vi "ReadStrains.vi"() -> ()   [LabVIEW 2017]
doc: "I. Description:\nThis example demonstrates how to make continuous, hardware-timed temperature measurement using a thermocouple.\n\nII. Instructions for Running:\n1. Specify the Physical Channel where you have connected the thermocouple.\n2. Enter the Minimum and Maximum temperature values in degrees C you expect to measure. A smaller range will allow a more accurate measurement.\n3. Enter the scan rate at which you want to run the acquisition.\n4. Specify the type of thermocouple you are using.\n5. Thermocouple measurements require cold-junction compensation (CJC) to correctly scale them. Specify the source of your cold-junction compensation.\n6. If your CJC source is \"Internal\", skip the rest of the steps.\n7. If your CJC source is \"Constant Value\", specify the value (usually room temperature) in degrees C.\n8. If your CJC source is \"Channel\", specify the CJC Channel name. \n9. Specify the appropriate Auto Zero Mode. See your device's hardware manual to find out if your device supports this attribute.\n\nIII. Block Diagram Steps:\n1. Create a Thermocouple (TC) temperature measurement channel.\n2. Get all the channels in the task.\n3. Convert channel(s) array to a comma-delimited channel string.\n4. This attribute is set to compensate for input offset errors. May not be supported by all devices*.\n5. Call the Timing VI to specify the hardware timing parameters. Use device's internal clock, continuous mode acquisition and the sample rate specified by the user.\n6. Call the Start VI to program and start the acquisition.\n7. Read N samples and plot it. By default, the Read VI reads all available samples, but you can specify how many samples to read at a time and the timeout value. Continue reading data until the stop button is pressed or an error occurs. \n8. Call the Clear Task VI to clear the Task.\n9. Use the popup dialog box to display an error if any.\n\n* If your device does not support Auto Zero Mode bypass Step 2, 3, and 4.\n\nIV. I/O Connections Overview:\nConnect your thermocouple to the terminals corresponding to the Physical Channel I/O Control value."
uses:
  <vilib>/Utility/error.llb/DialogType.ctl
  <vilib>/DAQmx/read.llb/DAQmx Read (Analog 1D Wfm NChan NSamp).vi
  <vilib>/Analysis/baseanly.llb/Mean (DBL).vi
  <vilib>/Waveform/WDTOps.llb/WDT Index Channel DBL.vi
  <vilib>/DAQmx/create/channels.llb/DAQmx Create Channel (AI-Voltage-Basic).vi
  <vilib>/DAQmx/configure/timing.llb/DAQmx Timing (Sample Clock).vi
  <vilib>/DAQmx/miscellaneous.llb/DAQmx Fill In Error Info.vi
  <vilib>/Analysis/NI_AALBase.lvlib
  <vilib>/ptbypt/NI_PtbyPt.lvlib
  <vilib>/Utility/miscctls.llb/LVRowAndColumnTypeDef.ctl
panel:
  in  "Data Tag":dbl=99.0 format="%.2p"
  out "Load Cell Min Peak":dbl format="%0.2f"
  out "Load Cell Max Peak":dbl format="%0.2f"
  in  "Stop":bool
  in  "Color Box":u32(colorbox)=16448250
  out "Results":i32[](listbox)
  in  "num_chans":i32=5
  out "TRQ_2SPD_OT (N·m)":dbl=-0.01305389404296875 format="%0.3f"
  out "Power_OT (W)":dbl=-4.779110606064606 format="%.2f"
  out "rpm_out/rpm_in":dbl=-8.382425226893735e-05 format="%.3g"
  out "AI Consumer Iterations":i32=456
  in  "path":path=path "D:/LabView Data"
  out "P2 - P1":dbl=2.2560862731933593 format="%.3f"
  out "Recorded Blocks":dbl=456.0
  in  "Force Record":bool caption="Force Record Enable"
  out "data 2":waveform(dbl)[](array[waveform])=[{"t0"=timestamp(3680889355.4831715 s since 1904-01-01), "dt"=0.001, "Y"=[-0.10400045911486416, -0.1030272812082663, -0.10335167384374958, -0.1030272812082663, -0.1030272812082663, -0.10270288857283233, -0.1030272812082663, -0.10270288857283233, -0.1030272812082663, -0.10367606647928221, -0.10335167384374958, -0.10367606647928221, -0.10367606647928221, -0.10367606647928221, -0.1072443854734039, -0.10237849593744763, -0.1030272812082663, -0.10270288857283233, -0.10432485175049552, -0.10367606647928221, -0.1030272812082663, -0.10335167384374958, -0.101729710666826, -0.10335167384374958, -0.10270288857283233, -0.1030272812082663, -0.10270288857283233, -0.1020541033021122, -0.10367606647928221, -0.10432485175049552, -0.10367606647928221, -0.10432485175049552, -0.10270288857283233, -0.10464924438617626, -0.10400045911486416, -0.10367606647928221, -0.10270288857283233, -0.10335167384374958, -0.1056224222935152, -0.10432485175049552, -0.10335167384374958, -0.1030272812082663, -0.10400045911486416, -0.1030272812082663, -0.10497363702190646, -0.10432485175049552, -0.10594681492939385, -0.09783699904722266, -0.10270288857283233, -0.10270288857283233, -0.10270288857283233, -0.10270288857283233, -0.10367606647928221, -0.10367606647928221, -0.10367606647928221, -0.10335167384374958, -0.10367606647928221, -0.10335167384374958, -0.10335167384374958, -0.1030272812082663, -0.10335167384374958, -0.10367606647928221, -0.10432485175049552, -0.10367606647928221, -0.10237849593744763, -0.10432485175049552, -0.1030272812082663, -0.10432485175049552, -0.10400045911486416, -0.10335167384374958, -0.10432485175049552, -0.101729710666826, -0.10335167384374958, -0.1030272812082663, -0.1020541033021122, -0.1030272812082663, -0.10270288857283233, -0.10400045911486416, -0.10432485175049552, -0.10627120756532199, -0.10367606647928221, -0.10400045911486416, -0.10237849593744763, -0.10432485175049552, -0.10367606647928221, -0.10367606647928221, -0.10237849593744763, -0.10400045911486416, -0.10756877810953042, -0.10400045911486416, -0.10237849593744763, -0.1030272812082663, -0.10270288857283233, -0.10335167384374958, -0.10335167384374958, -0.10432485175049552, -0.101729710666826, -0.10237849593744763, -0.1030272812082663, -0.10335167384374958, -0.10270288857283233, -0.10367606647928221, -0.10367606647928221, -0.10335167384374958, -0.1030272812082663, -0.10627120756532199, -0.1030272812082663, -0.10335167384374958, -0.10335167384374958, -0.1030272812082663, -0.10335167384374958, -0.1030272812082663, -0.10367606647928221, -0.10367606647928221, -0.1020541033021122, -0.10335167384374958, -0.1030272812082663, -0.10335167384374958, -0.10335167384374958, -0.10335167384374958, -0.10335167384374958, -0.10464924438617626, -0.101729710666826, -0.10270288857283233, -0.10270288857283233, -0.10270288857283233, -0.1030272812082663, -0.10270288857283233, -0.10497363702190646, -0.10756877810953042, -0.10400045911486416, -0.1030272812082663, -0.1030272812082663, -0.10367606647928221, -0.10335167384374958, -0.10400045911486416, -0.10367606647928221, -0.10432485175049552, -0.10627120756532199, -0.10497363702190646, -0.10335167384374958, -0.10367606647928221, -0.1030272812082663, -0.10335167384374958, -0.10400045911486416, -0.10335167384374958, -0.1095151339273331, -0.10432485175049552, -0.10335167384374958, -0.10237849593744763, -0.10335167384374958, -0.1030272812082663, -0.10432485175049552, -0.10270288857283233, -0.1030272812082663, -0.10756877810953042, -0.10270288857283233, -0.101729710666826, -0.10270288857283233, -0.1030272812082663, -0.10367606647928221, -0.10497363702190646, -0.10367606647928221, -0.1030272812082663, -0.1030272812082663, -0.10400045911486416, -0.10270288857283233, -0.10335167384374958, -0.1030272812082663, -0.10367606647928221, -0.10400045911486416, -0.09881017695146153, -0.101405318031589, -0.10270288857283233, -0.10270288857283233, -0.10367606647928221, -0.10400045911486416, -0.10367606647928221, -0.10367606647928221, -0.10627120756532199, -0.10367606647928221, -0.10367606647928221, -0.10270288857283233, -0.10237849593744763, -0.10464924438617626, -0.1030272812082663, -0.1030272812082663, -0.10335167384374958, -0.10627120756532199, -0.10464924438617626, -0.1030272812082663, -0.10270288857283233, -0.10270288857283233, -0.1030272812082663, -0.10367606647928221, -0.10400045911486416, -0.10075653276126252, -0.10400045911486416, -0.10270288857283233, -0.10335167384374958], "attributes"=variant("NI_ChannelName"=variant(string "Dev1/ai0"), "NI_UnitDescription"=variant(string "Volts"))}, {"t0"=timestamp(3680889355.4831853 s since 1904-01-01), "dt"=0.001, "Y"=[-0.090375968462633, -0.08972718319562067, -0.09005157582910267, -0.08972718319562067, -0.09005157582910267, -0.09005157582910267, -0.09005157582910267, -0.08972718319562067, -0.08972718319562067, -0.09005157582910267, -0.090375968462633, -0.09005157582910267, -0.090375968462633, -0.09070036109621166, -0.09297110953261792, -0.09102475372983868, -0.09070036109621166, -0.090375968462633, -0.09070036109621166, -0.09102475372983868, -0.090375968462633, -0.09005157582910267, -0.08940279056218697, -0.09005157582910267, -0.08972718319562067, -0.09005157582910267, -0.09005157582910267, -0.08940279056218697, -0.09005157582910267, -0.09070036109621166, -0.090375968462633, -0.09102475372983868, -0.090375968462633, -0.090375968462633, -0.09005157582910267, -0.09070036109621166, -0.09005157582910267, -0.09005157582910267, -0.09199793163101021, -0.0913491463635141, -0.09102475372983868, -0.090375968462633, -0.09070036109621166, -0.090375968462633, -0.09102475372983868, -0.0913491463635141, -0.09199793163101021, -0.08778082739574193, -0.08907839792880154, -0.08907839792880154, -0.08907839792880154, -0.08972718319562067, -0.090375968462633, -0.090375968462633, -0.09070036109621166, -0.09005157582910267, -0.09005157582910267, -0.090375968462633, -0.09005157582910267, -0.09005157582910267, -0.090375968462633, -0.09070036109621166, -0.09102475372983868, -0.09070036109621166, -0.090375968462633, -0.09070036109621166, -0.09005157582910267, -0.09070036109621166, -0.09070036109621166, -0.090375968462633, -0.09070036109621166, -0.08972718319562067, -0.090375968462633, -0.090375968462633, -0.08972718319562067, -0.09005157582910267, -0.08972718319562067, -0.09070036109621166, -0.09102475372983868, -0.09199793163101021, -0.09167353899723793, -0.09102475372983868, -0.090375968462633, -0.090375968462633, -0.090375968462633, -0.090375968462633, -0.08972718319562067, -0.090375968462633, -0.09264671689870017, -0.0913491463635141, -0.090375968462633, -0.090375968462633, -0.09005157582910267, -0.090375968462633, -0.09005157582910267, -0.09102475372983868, -0.08972718319562067, -0.08940279056218697, -0.09005157582910267, -0.09005157582910267, -0.08972718319562067, -0.08972718319562067, -0.09005157582910267, -0.09005157582910267, -0.090375968462633, -0.09167353899723793, -0.09070036109621166, -0.090375968462633, -0.090375968462633, -0.090375968462633, -0.090375968462633, -0.090375968462633, -0.09070036109621166, -0.09070036109621166, -0.09005157582910267, -0.08972718319562067, -0.08972718319562067, -0.08972718319562067, -0.08972718319562067, -0.090375968462633, -0.09005157582910267, -0.09102475372983868, -0.09005157582910267, -0.08972718319562067, -0.08972718319562067, -0.08972718319562067, -0.09005157582910267, -0.09005157582910267, -0.09070036109621166, -0.09264671689870017, -0.09167353899723793, -0.09102475372983868, -0.09005157582910267, -0.090375968462633, -0.09005157582910267, -0.09070036109621166, -0.090375968462633, -0.09070036109621166, -0.09167353899723793, -0.09232232426483095, -0.09102475372983868, -0.09070036109621166, -0.090375968462633, -0.09070036109621166, -0.09102475372983868, -0.09102475372983868, -0.09394428743466249, -0.09232232426483095, -0.0913491463635141, -0.09070036109621166, -0.090375968462633, -0.090375968462633, -0.09102475372983868, -0.09005157582910267, -0.09005157582910267, -0.09232232426483095, -0.0913491463635141, -0.09005157582910267, -0.09005157582910267, -0.08972718319562067, -0.090375968462633, -0.0913491463635141, -0.09070036109621166, -0.090375968462633, -0.09005157582910267, -0.09005157582910267, -0.09005157582910267, -0.09005157582910267, -0.08972718319562067, -0.09070036109621166, -0.09070036109621166, -0.08842961266217535, -0.08810522002893456, -0.08907839792880154, -0.08940279056218697, -0.09005157582910267, -0.09070036109621166, -0.09070036109621166, -0.090375968462633, -0.0913491463635141, -0.09102475372983868, -0.09070036109621166, -0.09005157582910267, -0.08972718319562067, -0.09070036109621166, -0.09005157582910267, -0.09005157582910267, -0.09005157582910267, -0.09199793163101021, -0.0913491463635141, -0.09102475372983868, -0.090375968462633, -0.09005157582910267, -0.09005157582910267, -0.090375968462633, -0.09070036109621166, -0.08907839792880154, -0.09005157582910267, -0.090375968462633, -0.09070036109621166], "attributes"=variant("NI_ChannelName"=variant(string "Dev1/ai1"), "NI_UnitDescription"=variant(string "Volts"))}, {"t0"=timestamp(3680889355.483199 s since 1904-01-01), "dt"=0.001, "Y"=[-0.1030272812082663, -0.1030272812082663, -0.10270288857283233, -0.10237849593744763, -0.10270288857283233, -0.10335167384374958, -0.10335167384374958, -0.10367606647928221, -0.10400045911486416, -0.10400045911486416, -0.10400045911486416, -0.10400045911486416, -0.10400045911486416, -0.10400045911486416, -0.10464924438617626, -0.10464924438617626, -0.10432485175049552, -0.10367606647928221, -0.10335167384374958, -0.10335167384374958, -0.10400045911486416, -0.10400045911486416, -0.10367606647928221, -0.10367606647928221, -0.10367606647928221, -0.10367606647928221, -0.10400045911486416, -0.10400045911486416, -0.10367606647928221, -0.10400045911486416, -0.10529802965768609, -0.10367606647928221, -0.10335167384374958, -0.1030272812082663, -0.10367606647928221, -0.10335167384374958, -0.10335167384374958, -0.10400045911486416, -0.10400045911486416, -0.10432485175049552, -0.10464924438617626, -0.10432485175049552, -0.10497363702190646, -0.10432485175049552, -0.10529802965768609, -0.10432485175049552, -0.10497363702190646, -0.10400045911486416, -0.1030272812082663, -0.1030272812082663, -0.10270288857283233, -0.10237849593744763, -0.10237849593744763, -0.1030272812082663, -0.1030272812082663, -0.10367606647928221, -0.10367606647928221, -0.10400045911486416, -0.10400045911486416, -0.10464924438617626, -0.10464924438617626, -0.10464924438617626, -0.10400045911486416, -0.10432485175049552, -0.10400045911486416, -0.10400045911486416, -0.10335167384374958, -0.10335167384374958, -0.10335167384374958, -0.1030272812082663, -0.10367606647928221, -0.10400045911486416, -0.1030272812082663, -0.10367606647928221, -0.10367606647928221, -0.10400045911486416, -0.10367606647928221, -0.10497363702190646, -0.10432485175049552, -0.10529802965768609, -0.10432485175049552, -0.10464924438617626, -0.10400045911486416, -0.10335167384374958, -0.10335167384374958, -0.10367606647928221, -0.10335167384374958, -0.10400045911486416, -0.10400045911486416, -0.10464924438617626, -0.10432485175049552, -0.10497363702190646, -0.10432485175049552, -0.10432485175049552, -0.10464924438617626, -0.10400045911486416, -0.10400045911486416, -0.10400045911486416, -0.10335167384374958, -0.10335167384374958, -0.1030272812082663, -0.1030272812082663, -0.1030272812082663, -0.10270288857283233, -0.1030272812082663, -0.10367606647928221, -0.10367606647928221, -0.10400045911486416, -0.10400045911486416, -0.10432485175049552, -0.10464924438617626, -0.10400045911486416, -0.10400045911486416, -0.10432485175049552, -0.10367606647928221, -0.10335167384374958, -0.10335167384374958, -0.1030272812082663, -0.10335167384374958, -0.10270288857283233, -0.10270288857283233, -0.10367606647928221, -0.10400045911486416, -0.10367606647928221, -0.10432485175049552, -0.10432485175049552, -0.10335167384374958, -0.10432485175049552, -0.10464924438617626, -0.1056224222935152, -0.10464924438617626, -0.10464924438617626, -0.10400045911486416, -0.10335167384374958, -0.10335167384374958, -0.10335167384374958, -0.10270288857283233, -0.10367606647928221, -0.10400045911486416, -0.10464924438617626, -0.10497363702190646, -0.10497363702190646, -0.10497363702190646, -0.10400045911486416, -0.10529802965768609, -0.10464924438617626, -0.1056224222935152, -0.1056224222935152, -0.10464924438617626, -0.10497363702190646, -0.10432485175049552, -0.10464924438617626, -0.10367606647928221, -0.10335167384374958, -0.10367606647928221, -0.10464924438617626, -0.10432485175049552, -0.10432485175049552, -0.10432485175049552, -0.10400045911486416, -0.10400045911486416, -0.10464924438617626, -0.10432485175049552, -0.10464924438617626, -0.10367606647928221, -0.10335167384374958, -0.1030272812082663, -0.10335167384374958, -0.10335167384374958, -0.10335167384374958, -0.10367606647928221, -0.1030272812082663, -0.1030272812082663, -0.10270288857283233, -0.10335167384374958, -0.10270288857283233, -0.10335167384374958, -0.10367606647928221, -0.10432485175049552, -0.10432485175049552, -0.10497363702190646, -0.10432485175049552, -0.10367606647928221, -0.10335167384374958, -0.10432485175049552, -0.10335167384374958, -0.10335167384374958, -0.10335167384374958, -0.10400045911486416, -0.10432485175049552, -0.10464924438617626, -0.10464924438617626, -0.10367606647928221, -0.10400045911486416, -0.10464924438617626, -0.10400045911486416, -0.10367606647928221, -0.10432485175049552, -0.10335167384374958, -0.10270288857283233], "attributes"=variant("NI_ChannelName"=variant(string "Dev1/ai2"), "NI_UnitDescription"=variant(string "Volts"))}, {"t0"=timestamp(3680889355.4832134 s since 1904-01-01), "dt"=0.001, "Y"=[9.970761347134479, 9.980493438515435, 10.057052580026493, 10.050240112411151, 10.024287857756553, 9.963948883552924, 10.009689716548086, 9.985683887516803, 9.9600560473629, 9.977573811033155, 9.974654183609161, 9.938645450165463, 9.976276198837517, 9.89614866799873, 9.958758435322546, 9.986657096725082, 10.014880166587908, 10.06808229017756, 10.063216241478031, 10.057052580026493, 10.042454435528043, 10.031100324154862, 10.03207353366638, 10.014880166587908, 9.993793964450594, 10.021043826250418, 9.967841719846424, 9.942538285787142, 9.947728733443315, 9.958434032314253, 9.952270375293104, 9.973356571439426, 10.001904041834917, 10.023963454602686, 9.984710678315004, 10.021368229397778, 10.057701386482737, 10.020395019957865, 10.040832419563271, 10.016502182263276, 9.995415979891405, 9.967517316818013, 9.966868510763346, 9.953892390273543, 9.919181273604169, 9.97173455624344, 9.920154482371043, 9.957785226299821, 9.969139331967257, 10.004499266693117, 9.996064786072774, 9.987305902867535, 10.059972209102451, 10.035966371777608, 10.032722340011015, 10.057376983254251, 10.022017035694667, 9.998011204634192, 9.979844632403223, 9.942862688760275, 9.925344929236438, 9.91723485608973, 9.96200246544498, 9.92891336156266, 9.980493438515435, 9.995415979891405, 10.006445685367076, 10.03207353366638, 10.04180562913996, 10.087870889907263, 10.03499316224003, 10.053159741349983, 9.93637462943381, 10.006121282252945, 9.980169035458967, 10.00352605736588, 9.965570898662637, 9.928264555678723, 9.949350748373524, 9.960704853387385, 9.945133509592281, 9.972707765358873, 9.99963322012187, 10.022017035694667, 10.052186531697178, 10.0512133220509, 10.06126982204397, 10.038237194057304, 10.040832419563271, 10.035966371777608, 10.00255284804514, 10.000606429423135, 9.929562167449461, 9.968814928935972, 9.933779405783481, 9.966219704711555, 9.937347838314507, 9.958758435322546, 9.976600601885348, 10.007418894713798, 10.036939581321704, 10.024287857756553, 10.052186531697178, 10.040832419563271, 10.033695549533391, 10.043752048312902, 10.017475391677165, 9.976925004933896, 9.972707765358873, 9.963948883552924, 9.95356798727602, 9.930535376285032, 9.987630305939843, 9.942213882814727, 9.978547020187436, 9.984386275249179, 9.99768680153882, 10.062243031757733, 10.047320483531054, 10.051862128481027, 10.02169263254586, 10.042454435528043, 9.96427328657343, 10.018773004239138, 9.977898214083861, 9.98146664768915, 9.97303216839879, 9.951297166313452, 9.938645450165463, 9.957136420288261, 9.937023435353558, 9.973356571439426, 9.992171949027805, 9.993469561364593, 10.02915390515136, 10.057701386482737, 10.071975129254877, 10.03629077495825, 10.053159741349983, 10.038237194057304, 10.01844860109756, 9.970112541065435, 9.933130599878064, 9.98081784157262, 9.942862688760275, 9.972058959281199, 9.943511494708691, 9.951621569305953, 9.978871423240303, 9.998011204634192, 9.976925004933896, 9.983413066056023, 10.069379903191706, 10.04537406431028, 10.04991570919935, 10.04796928994378, 10.015528972855886, 10.014231360322817, 9.997362398444167, 9.954541196270744, 9.95032395734026, 9.919830079448037, 9.96200246544498, 9.952919181283127, 9.972058959281199, 9.992820755194758, 10.029802711482967, 10.055754967122715, 10.006445685367076, 10.051862128481027, 10.02363905144954, 10.038561597243016, 10.057701386482737, 10.014880166587908, 9.972058959281199, 9.959082838331556, 10.037588387688057, 9.927291346858187, 9.929886570393936, 9.926642540981407, 9.92339851164045, 9.960380450374785, 9.987954709012872, 10.017475391677165, 10.019097407381437, 10.058025789711948, 10.067109080424581, 10.02688308301353, 9.956812017283559, 10.046347273917407, 10.015204569721535, 9.986008290585508, 9.950648360330606, 9.98146664768915, 9.923074108710292, 9.96524649563926, 9.932481793975509, 9.956487614279574, 9.983088662993078, 10.021368229397778], "attributes"=variant("NI_ChannelName"=variant(string "Dev1/ai3"), "NI_UnitDescription"=variant(string "Volts"))}]
  out "Power_IN (W)":dbl=0.0005711775684961294 format="%.2g"
  out "TRQ_2SPD_DRVLN_OT (N·m)":dbl=-0.018612060546874976 format="%0.3f"
  out "Waveform Chart":waveform(dbl)[](graph)=[{"t0"=timestamp(3680889355.4831715 s since 1904-01-01), "dt"=0.01, "Y"=[-20.631407652497842, -20.75467685406648, -20.59896838896825, -20.780628264870508, -20.637895505396592, -20.663846916046168, -20.728725443162563, -20.696286179664597, -20.793603970347206, -20.59248053625661, -20.709261885055327, -20.644383357919143, -20.722237590555686, -20.806579675725974, -20.806579675853744, -20.683310474277953, -20.70277403231996, -20.618431947232246, -20.748189001336023, -20.598968388981042], "attributes"=variant("NI_ChannelName"=variant(string "HS_LOADCELL_A_LBF"), "NI_UnitDescription"=variant(string "lbf"))}, {"t0"=timestamp(3680889355.4831853 s since 1904-01-01), "dt"=0.01, "Y"=[-17.99085160781258, -18.16602362995864, -17.99733946048705, -18.12709651391563, -18.055730134580486, -18.01680301849887, -18.114120808557974, -18.088169397890056, -18.16602362996153, -18.029778723839122, -18.068705839868564, -18.029778723838152, -18.075193692560465, -18.1789993353008, -18.26334142007583, -18.107632955909622, -18.068705839864695, -17.977875902519663, -18.114120808576352, -18.05573013452541], "attributes"=variant("NI_ChannelName"=variant(string "HS_LOADCELL_B_LBF"), "NI_UnitDescription"=variant(string "lbf"))}, {"t0"=timestamp(3680889355.483199 s since 1904-01-01), "dt"=0.01, "Y"=[-0.10322191678961545, -0.1040004591149086, -0.10383826279707317, -0.10380582353359895, -0.10429241248705587, -0.10335167384387292, -0.10387070206069556, -0.10403289837852114, -0.10393558058779713, -0.10413021616916611, -0.10344899163446859, -0.10364362721580296, -0.10406533764211885, -0.10383826279716202, -0.1049736370219559, -0.10413021616915127, -0.10377338427002589, -0.10341655237092517, -0.10390314132425375, -0.1039680198513899], "attributes"=variant("NI_ChannelName"=variant(string "HS_2210_STRAIN_B_VOLTS"), "NI_UnitDescription"=variant(string "V"))}, {"t0"=timestamp(3680889355.4832134 s since 1904-01-01), "dt"=0.01, "Y"=[9.997978768185797, 9.993437131092849, 9.995188902202935, 10.009300435915007, 9.962618833492515, 10.0112144154578, 9.987760076882132, 9.981823496420388, 10.021919719195791, 9.968166125458495, 10.016275103370784, 9.993599329306088, 9.982666942582545, 10.01825396484399, 9.96894469235443, 10.015464096552865, 9.989382089044614, 9.988733284529754, 10.006348371443773, 9.97150747733223], "attributes"=variant("NI_ChannelName"=variant(string "HS_2210_EXC_VOLTS"), "NI_UnitDescription"=variant(string "V"))}]
  in  "Run Letter":string="a"
  out "Recording":bool
  in  "Num_Blocks":dbl=100.0
  in  "Maximum Value":dbl=10.0 format="%0.2f"
  in  "Minimum Value":dbl=-10.0 format="%0.2f"
  in  "Physical Channel":tag="Dev1/ai0:4" caption="PCI-6143_1 Channels"
  in  "Rate":dbl=10.0 format="%0.2f"
  # "rev 150415_A  added \"Record Run X\" sub VI.\nrev 150423_A added power, efficiency, and manual inputs for speed .\nrev 150423_B added speed measurement via PCI-6602 card.\nrev 161117_A is set up for the alternator test reading shaft RPM from Dynapar encoder and torque from the Omega TQ513-1K paired with the Omega DP41-S.\nrev 170504_A migrated DAQ h/w from the SCXI chassis (now being used for TC2 porcupine testing) to PCI-6143.\nrev 170510_A takes data at 1000Hz, then averages groups of 100 samples for a logging rate of 10Hz per channel.  Added function that resets \"Data Tag\"\nto 99 after \"Num_Blocks\" has been recorded.\nrev 170810_A adds flowmeter for 2-speed supercharger drive bench test.  CJP\nrev 170821_A logs tags to same file for a given run letter.  Uses \"Record Continuous Tags...\" sub VI.\nrev 171129_A is for the Orthrus 2-speed drive.  Added new encoder period measurement for the 127 tooth geat \"RPM_2SPD_OT\". CJP\nrev 171130_A adds Digital Output (DO) for 2SPD drive control.  Will log this with the rest of the data.  Also corrected the number of teeth on the 2SPD Output side from 127 to 107!\nrev 171201_A restructuring for  \"real-time\" response to speed changes by moving the disklog to a separate loop (queue).\nrev 171201_B moves counters into main AI loop and adds a start trigger so DAQ won't start until rig is spinning.  Added F-V where old \"F1\" channel was for \"RPM_2SPD_OT\".   CJP\nrev 171201_C uses a CI-Frequency task for RPM instead of period.  Testing this for better transient response.  This appears to be even slower than the period measurement.\nrev 171201_D is built from rev 171201_A, but adding in the F-V channel.  This version queues both the AI channel and CI channels to a single Consumer.  Also adding a 30s switch to automate switching of the 2SPD solenoid.\nrev 171221_A was the first attempt at this and for some reason, while running that VI, the computer froze, unable to do ctrl+alt+del reboot.  After rebooting, the VI was no longer openable in LabView 2014 or LabView 2016.  Will try the same process over with v171226_A.\nrev 171226_A adds one more PCI_6143 card for 8 additional analog inputs.\nrev 171226_B created a backup with 171226_A.\nrev 180314_A added thermocouple for Sumanth.  This is for testing the 2-Speed Drive.\nrev Read \"ThermVolt_TestSpeed_180406_A.vi\" is for verifying the one remaining Micro-Epsilon speed sensor on the 2Spd Drive.\nrev \"Read Thermocouples and Voltages v180406_A.vi\" reintroduces the two counter/timer channels on the PCI-6602 card for the driveline encoder and \nMicro-Epsilon 2Spd Output.\nrev 180919_A built off of rev 180426_A for 2-Speed Drive testing.  CJP\nv181002_A adding new T22 at 2SPD input pulley AND keeping original T22 at output end of drivline.  CJP\nv181004_A corrected front panel displays for Power_IN and Power_OT.  CJP\nv181025_A adding ReadChnCfg.VI to read channel names, units, scaling, and offset from Labview Channel Map\nv190401_A restructuring \"Read Thermocouples and Voltages...\" to use only channels from NI-6229 out of test cell 2.  CJP\nv190516_A adds frequency measurement for driveline speed since F-V measurements not working.  CJP"
  # "For instructions, select Help>>Show Context Help"
  # "Now using 360 PPR encoder for input speed 171227.\nChanged to Input Gear Speed 180118.  CJP  127 Hz = 1 RPS, 127 Hz = 60 RPM\n5 kHz = 1 V => 5000/127 = 39.37 RPS = 2362.205 RPM\nv180314_A 5kHz = 1V = 5000/360 = 13.888 RPS = 833.33 RPM.\nBack to 360PPR encoder with pulley ratio of 1.48."
  # "HBM T21WN"
  # "Interface T22"
  # "Timing Parameters"
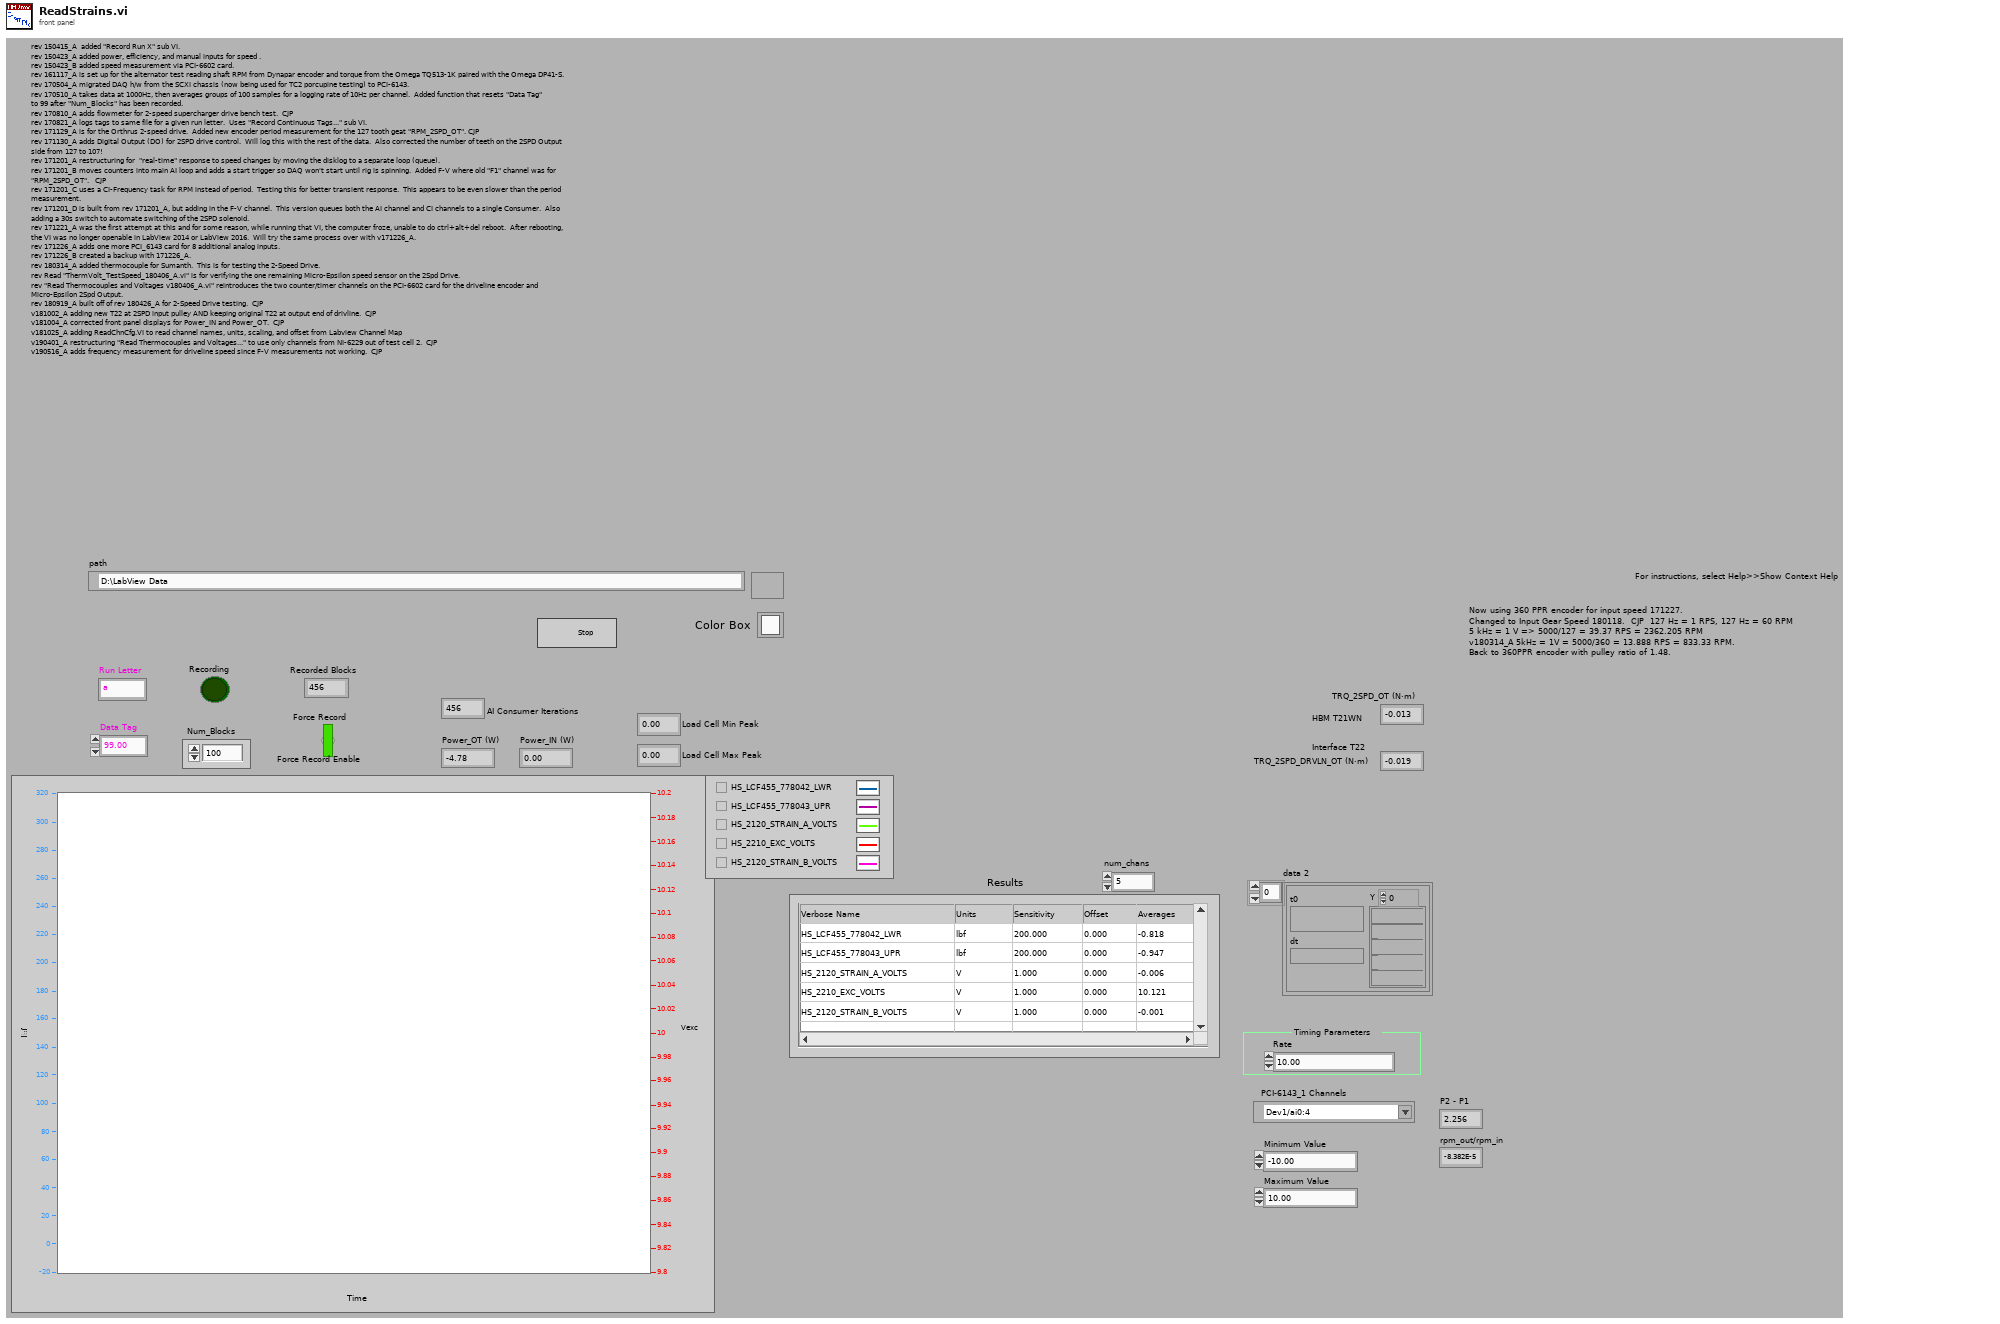
[diagram p1: front panel]
types:
  T1 = typedef "DialogType.ctl" = u16
  T2 = typedef "LVRowAndColumnTypeDef.ctl" = cluster{"Row":i32, "Column":i32}
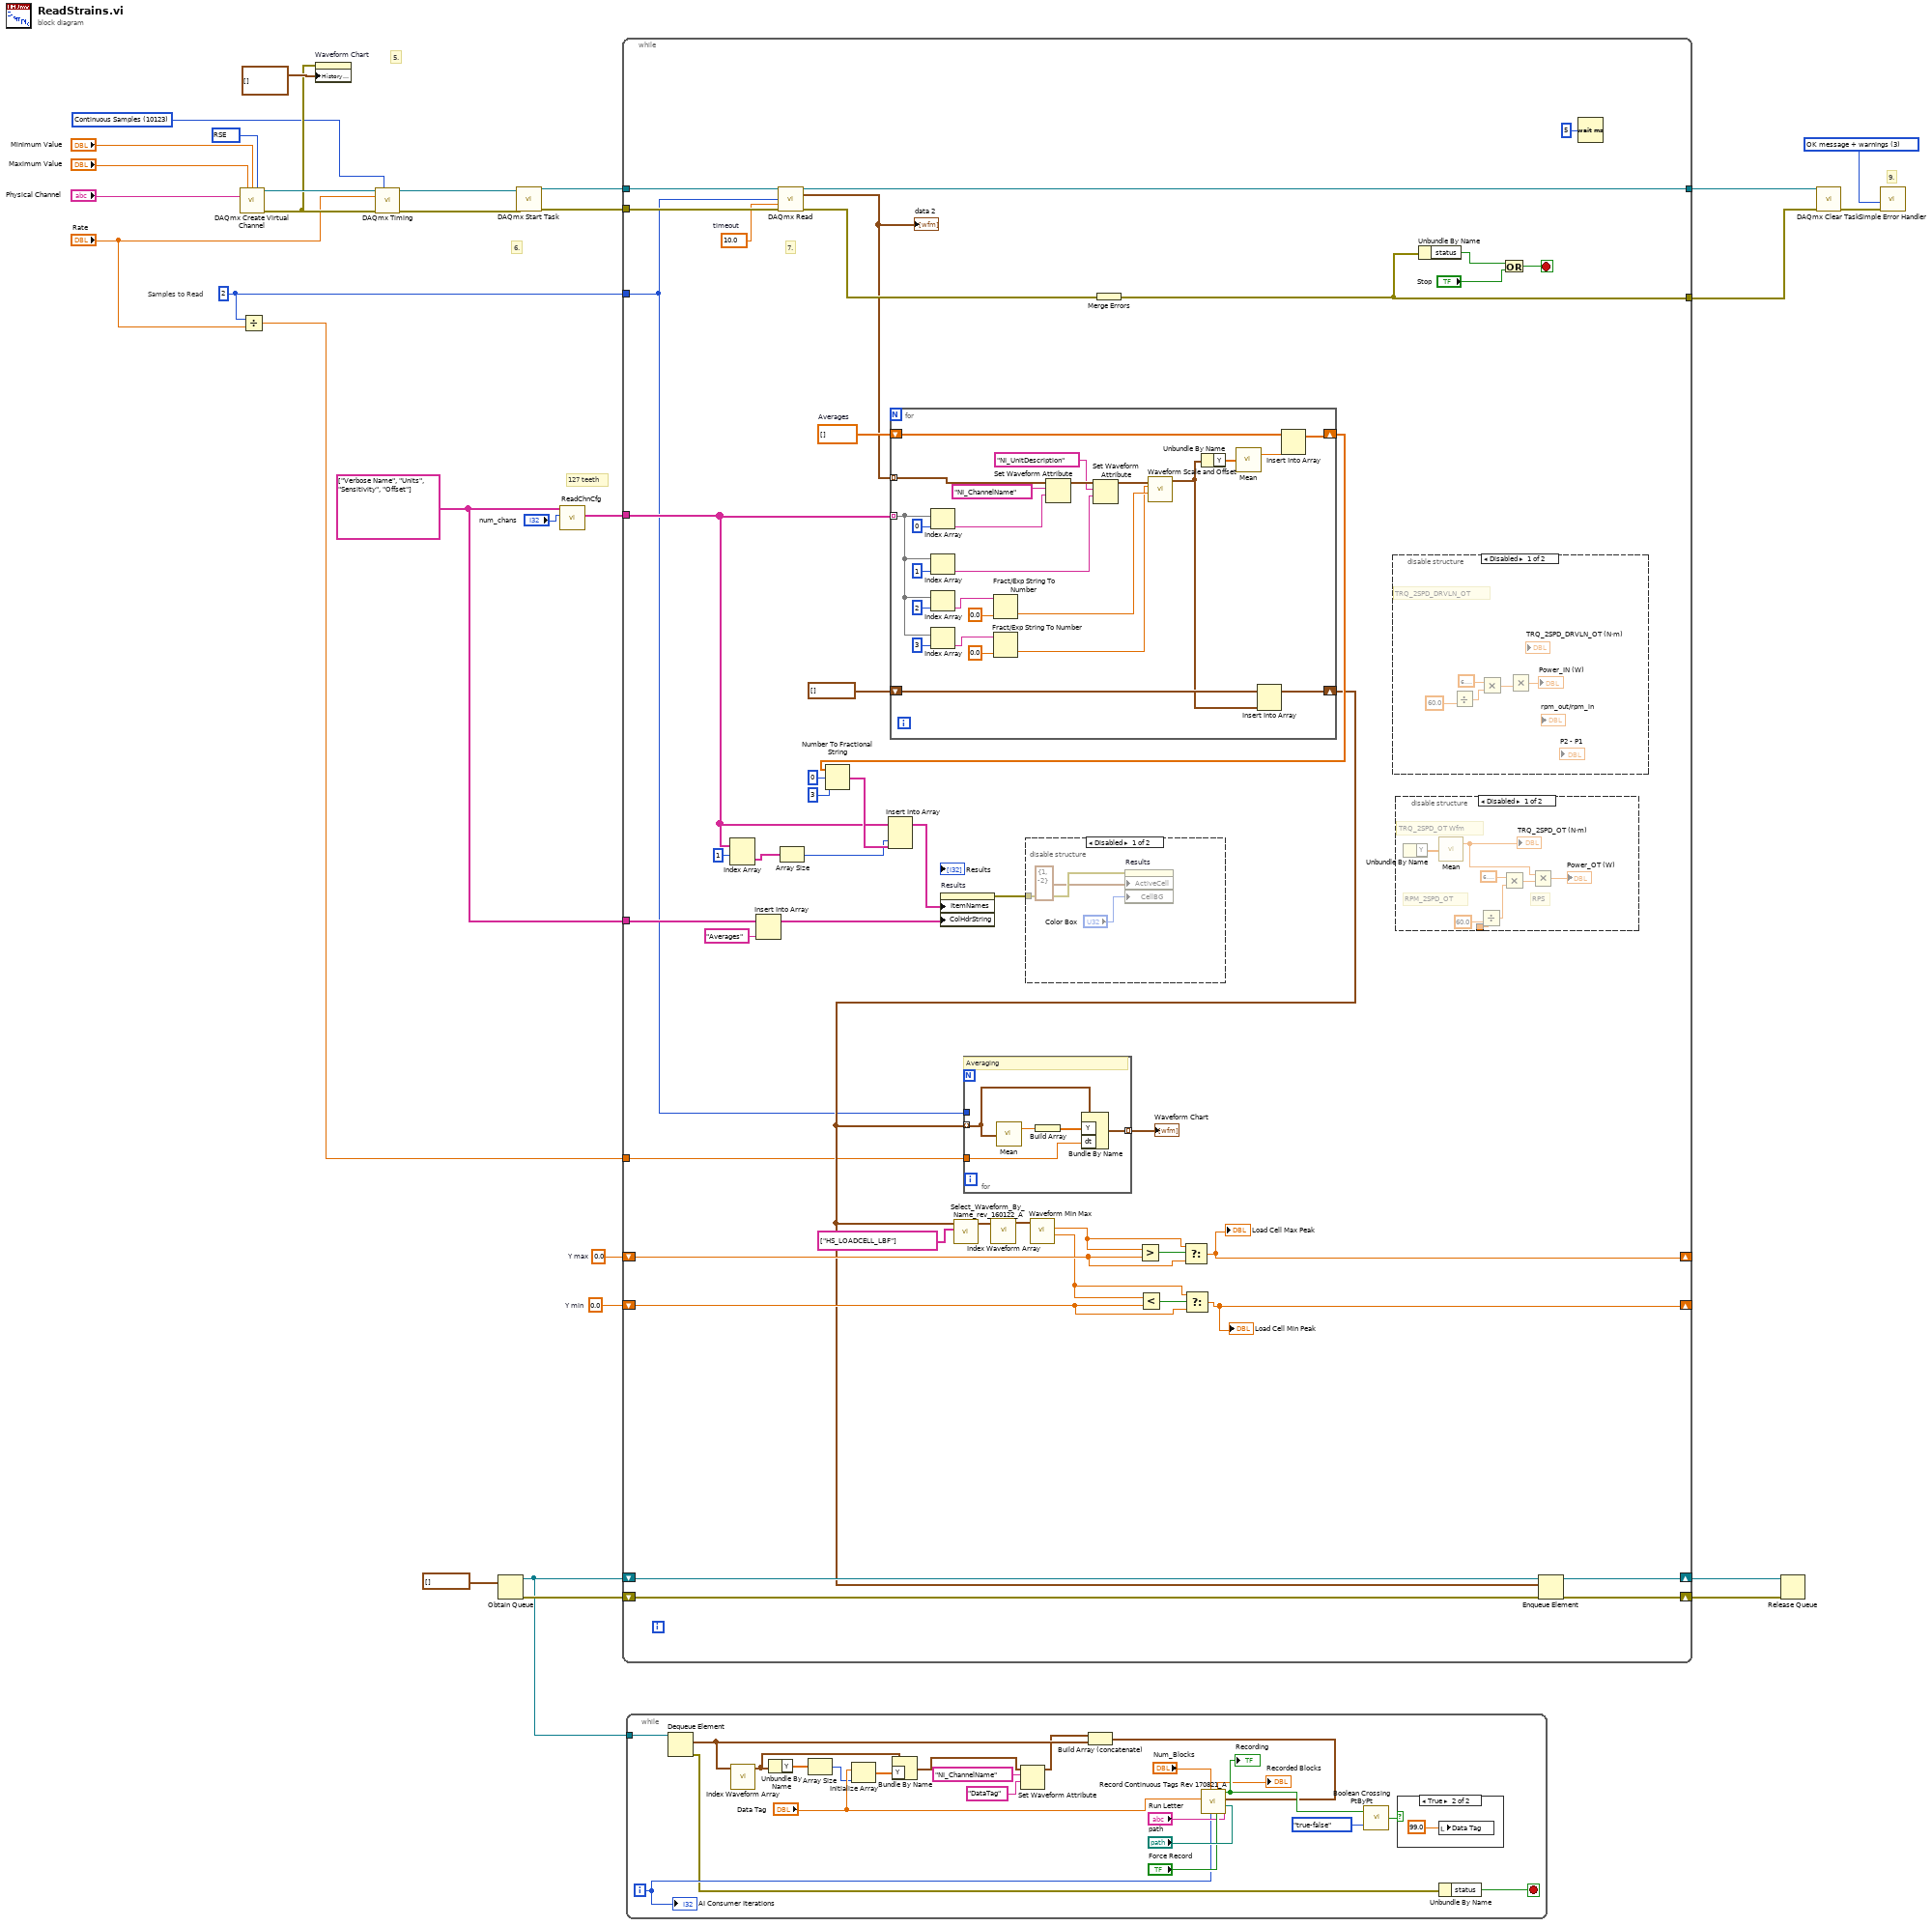
[diagram p0: block diagram]
diagram:
  w9 = string[] ["Verbose Name", "Units", "Sensitivity", "Offset"] ("Search Strings")
  w4 = 0.0  # Y min
  w5 = 0.0  # Y max
  w6 = 10083 items=["Default"=-1, "RSE"=10083, "NRSE"=10078, "Differential"=10106, "Pseudodifferential"=12529] ("input terminal configuration")
  w3 = 2 ("number of samples per channel")
  w24 = T1 3 items=["no dialog", "OK message", "continue or stop message", "OK message + warnings", "continue/stop + warnings"] ("type of dialog (OK msg:1)")
  w12 = 10123 items=["Finite Samples"=10178, "Continuous Samples"=10123] ("sample mode")
  # "127 teeth"
  # "Samples to Read"
  # "9."
  # "5."
  # "6."
  n1 = call-poly <vilib>:"DAQmx Create Virtual Channel.vi"("maximum value"="Maximum Value", "minimum value"="Minimum Value", "input terminal configuration"=w6, "physical channels"="Physical Channel") -> ("task out"=w22:refnum<k21>, "error out"=w20:errorcluster)  [unwired: 10 in]
  n2 = Divide(x=w3, y="Rate") -> (x/y=w2:dbl)
  n3 = property on="Waveform Chart" class="WFChart (strict)"(error in=w20, "History Data"=waveform(dbl)[][] []) -> ()  [unwired: 1 in, 2 out]
  n4 = call-poly <vilib>:"DAQmx Timing.vi"("task/channels in"=w22, "sample mode"=w12, "rate"="Rate", "error in"=w20) -> ("task out"=w25:refnum<k21>, "error out"=w7:errorcluster)  [unwired: 10 in]
  n5 = Obtain Queue(element data type=waveform(dbl)[] [] ("appended array")) -> (queue out=w15:refnum<queue>, error out=w18:errorcluster)  [unwired: 4 in, 1 out]
  n6 = call <vilib>:"DAQmx Start Task.vi"("task/channels in"=w25, "error in"=w7) -> ("task out"=w27:refnum<k21>, "error out"=w28:errorcluster)  [unwired: 12 in]
  n7 = call "ReadChnCfg.vi"("num_chans"="num_chans", "Search Strings"=w9) -> ("Table Minus Headers"=w10:string[][])  [unwired: 8 in, 1 out]
  n8 = while {
    tunnel: w27 -> [w74]
    tunnel: w28 -> [w73]
    tunnel: [w72] -> w26
    tunnel: w3 -> [w31]
    shift-right: [w65] -> w17
    shift-left: w15 -> [w67]
    shift-right: [w64] -> w16
    shift-left: w18 -> [w66]
    tunnel: [w48] -> w8
    tunnel: w10 -> [w51]
    tunnel: w9 -> [w61]
    shift-right: [w37] -> _
    shift-left: w5 -> [w38]
    shift-right: [w34] -> _
    shift-left: w4 -> [w33]
    tunnel: w2 -> [w30]
    stop <- w69 stop-if-true
    w63 = dbl[] []  # Averages
    w70 = 10.0  # timeout
    # "7."
    n9 = Index Array(array=w51, index (row)=1) -> (element=w55:string[])  [unwired: 1 in]
    n10 = Insert Into Array(array=w61, new element="Averages" ("new element/subarray")) -> (w52:string[])  [unwired: 1 in]
    n11 = call-poly <vilib>:"DAQmx Read.vi"("task/channels in"=w74, "number of samples per channel"=w31, "timeout"=w70, "error in"=w73) -> ("task out"=w72:refnum<k21>, "data"=w45:waveform(dbl)[], "error out"=w49:errorcluster)  [unwired: 9 in]
    "data 2" <- w45
    n12 = Array Size(array=w55) -> (size(s)=w54:i32)
    n13 = for {
      tunnel: w45 -> [w107] mode=indexing
      shift-right: [w106] -> w46
      shift-left: w63 -> [w105]
      tunnel: w51 -> [w94] mode=indexing
      shift-right: [w101] -> w32
      shift-left: waveform(dbl)[] [] -> [w103]
      n14 = Index Array(array=w94, index=0) -> (element=w98:string)
      n15 = Index Array(array=w94, index=1) -> (element=w97:string)
      n16 = Index Array(array=w94, index=2) -> (element=w93:string)
      n17 = Index Array(array=w94, index=3) -> (element=w89:string)
      n18 = Fract/Exp String To Number(string=w93, default (0 dbl)=0.0) -> (number=w91:dbl)  [unwired: 2 in, 1 out]
      n19 = Fract/Exp String To Number(string=w89, default (0 dbl)=0.0) -> (number=w88:dbl)  [unwired: 2 in, 1 out]
      n20 = Set Waveform Attribute(5:w98, 6:"NI_ChannelName" ("name"), 7:w107) -> (3:w111:waveform(dbl))  [unwired: 1 in, 2 out]
      n21 = Set Waveform Attribute(5:w97, 6:"NI_UnitDescription" ("name"), 7:w111) -> (3:w109:waveform(dbl))  [unwired: 1 in, 2 out]
      n22 = call <vilib>:"Waveform Scale and Offset.vi"("scale"=w91, "offset"=w88, "waveform in"=w109) -> ("waveform out"=w102:waveform(dbl))  [unwired: 7 in, 1 out]
      n23 = Unbundle By Name(w102) -> ("Y"=w108:dbl[])
      n24 = call-poly <vilib>:"Mean.vi"("X"=w108) -> ("mean"=w104:dbl)  [unwired: 1 out]
      n25 = Insert Into Array(array=w103, new element=w102) -> (w101:waveform(dbl)[])  [unwired: 1 in]
      n26 = Insert Into Array(array=w105, new element=w104) -> (w106:dbl[])  [unwired: 1 in]
    }
    n27 = Number To Fractional String(number=w46, width (-)=i16 0, precision (6)=i16 3) -> (F-format string=w57:string[])  [unwired: 1 in]
    n28 = Insert Into Array(array=w51, index (col)=w54, new element=w57) -> (w53:string[][])  [unwired: 1 in]
    n29 = property on="Results" class="MCListbox (strict)"("ItemNames"=w53, "ColHdrString"=w52) -> (error out=w50:errorcluster)  [unwired: 2 in, 1 out]
    n30 = call "Select_Waveform_By_Name_rev_160122_A.vi"("Array"=string[] ["HS_LOADCELL_LBF"], "Waveform Array"=w32) -> ("Array 2"=w42:waveform(dbl)[])  [unwired: 9 in]
    n31 = for {
      tunnel: w32 -> [w81] mode=indexing
      tunnel: [w82] -> w44 mode=indexing
      tunnel: w31 -> [_]
      tunnel: w30 -> [w78]
      # "Averaging"
      n32 = call-poly <vilib>:"Mean.vi"("X"=w81) -> ("mean"=w80:dbl)  [unwired: 1 out]
      n33 = Build Array(w80) -> (w79:dbl[])
      n34 = Bundle By Name(cluster=w81, "Y"=w79, "dt"=w78) -> (w82:waveform(dbl))
    }
    "Waveform Chart" <- w44
    n35 = call-poly <vilib>:"Index Waveform Array.vi"("waveform array"=w42) -> ("waveform"=w41:waveform(dbl))  [unwired: 9 in, 1 out]
    n36 = disable-structure shown="Disabled" {
      disable-tunnel: w50 -> [w77 _]
      frame Disabled {
        n37 = property on="Results" class="MCListbox (strict)"(error in=w77, "ActiveCell"=T2 {"Row"=1, "Column"=-2} ("Active Cell:Active Cell"), "CellBG"="Color Box") -> ()  [unwired: 1 in, 2 out]
      }
      frame Enabled {
      }
    }
    n38 = call <vilib>:"Waveform Min Max.vi"("waveform in"=w41) -> ("Y min"=w35:dbl, "Y max"=w39:dbl)  [unwired: 5 in, 4 out]
    n39 = Merge Errors(w49) -> (w48:errorcluster)
    n40 = Greater?(x=w39, y=w38) -> (0:w40:bool)
    n41 = Less?(x=w35, y=w33) -> (x < y?=w36:bool)
    n42 = Select(t=w39, s=w40, f=w38) -> (s? t:f=w37:dbl)
    "Load Cell Max Peak" <- w37
    n43 = Select(t=w35, s=w36, f=w33) -> (s? t:f=w34:dbl)
    "Load Cell Min Peak" <- w34
    n44 = disable-structure shown="Disabled" {
      frame Disabled {
        # "TRQ_2SPD_DRVLN_OT"
        n45 = Divide(y=60.0) -> (x/y=w83:dbl)  [unwired: 1 in]
        n46 = Multiply(x=6.283185307179586, y=w83) -> (x*y=w86:dbl)
        n47 = Multiply(y=w86) -> (x*y=→"Power_IN (W)":dbl)  [unwired: 1 in]
      }
      frame Enabled {
      }
    }
    n48 = disable-structure shown="Disabled" {
      disable-tunnel: _ -> [w113 _]
      frame Disabled {
        # "RPM_2SPD_OT"
        # "TRQ_2SPD_OT Wfm"
        # "RPS"
        n49 = Unbundle By Name() -> ("Y"=w117:dbl[])  [unwired: 1 in]
        n50 = call-poly <vilib>:"Mean.vi"("X"=w117) -> ("mean"=w116:dbl)  [unwired: 1 out]
        "TRQ_2SPD_OT (N·m)" <- w116
        n51 = Divide(x=w113, y=60.0) -> (x/y=w114:dbl)
        n52 = Multiply(x=6.283185307179586, y=w114) -> (x*y=w119:dbl)
        n53 = Multiply(x=w116, y=w119) -> (x*y=→"Power_OT (W)":dbl)
      }
      frame Enabled {
      }
    }
    n54 = Unbundle By Name(w48) -> ("status"=w71:bool)
    n55 = Or(x=w71, y="Stop") -> (x .or. y?=w69:bool)
    n56 = Enqueue Element(queue=w67, element=w32, error in (no error)=w66) -> (queue out=w65:refnum<queue>, error out=w64:errorcluster)  [unwired: 1 in, 1 out]
    n57 = Wait (ms)(milliseconds to wait=u32 5) -> ()  [unwired: 1 out]
  }
  n58 = while {
    tunnel: w15 -> [w135]
    i -> [w134]
    stop <- w132 stop-if-true
    n59 = Dequeue Element(queue=w135) -> (element=w123:waveform(dbl)[], error out=w133:errorcluster)  [unwired: 2 in, 2 out]
    n60 = call-poly <vilib>:"Index Waveform Array.vi"("waveform array"=w123) -> ("waveform"=w127:waveform(dbl))  [unwired: 9 in, 1 out]
    n61 = Unbundle By Name(w127) -> ("Y"=w131:dbl[])
    n62 = Array Size(array=w131) -> (size(s)=w129:i32)
    n63 = Initialize Array("Data Tag", w129) -> (w128:dbl[])
    n64 = Bundle By Name(cluster=w127, "Y"=w128) -> (w126:waveform(dbl))
    n65 = Set Waveform Attribute(5:"DataTag" ("name"), 6:"NI_ChannelName" ("name"), 7:w126) -> (3:w122:waveform(dbl))  [unwired: 1 in, 2 out]
    n66 = Build Array (concatenate)(w122, w123) -> (w121:waveform(dbl)[])
    n67 = call "Record Continuous Tags Rev 170821_A.vi"("Run Letter"="Run Letter", "path"="path", "Waveform Array In"=w121, "Force Record"="Force Record", "Main Count"=w134, "Num_Blocks"="Num_Blocks", "Data Tag"="Data Tag") -> ("Record Cmd"=w141:bool, "Recorded Blocks"=→"Recorded Blocks":dbl)  [unwired: 2 in, 1 out]
    "Recording" <- w141
    n68 = call <vilib>:"Boolean Crossing PtByPt.vi"("direction"=enum16{"either", "false-true", "true-false"}."true-false", "input"=w141) -> ("crossing"=w142:bool)  [unwired: 1 in]
    n69 = case shown="True" w142 {
      frame False {
      }
      frame True {
        n70 = local write "Data Tag"(99.0 ("y")) -> ()
      }
    }
    n71 = Unbundle By Name(w133) -> ("status"=w132:bool)
    "AI Consumer Iterations" <- w134
  }
  n72 = Release Queue(queue=w17, error in (no error)=w16) -> ()  [unwired: 1 in, 3 out]
  n73 = call <vilib>:"DAQmx Clear Task.vi"("task in"=w26, "error in"=w8) -> ("error out"=w29:errorcluster)  [unwired: 13 in]
  n74 = call <vilib>:"Simple Error Handler.vi"("type of dialog (OK msg:1)"=w24, "error in (no error)"=w29) -> ()  [unwired: 3 in, 5 out]
